vi "WIP_Read_Queue.vi"(8 "error in (no error)":errorcluster, 11 "Queue In":refnum<queue>) -> (0 "error out":errorcluster, 1 "State Out[]":T1[](array[typedef]), 2 "State Out":T1, 3 "Queue out":refnum<queue>)   [LabVIEW 2020]
uses:
  Controls/WIP_State.ctl
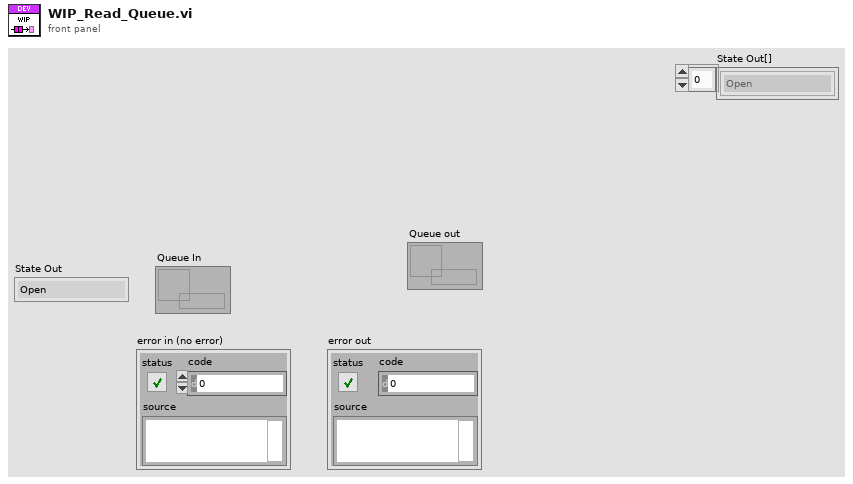
[diagram p1: front panel]
types:
  T1 = typedef "WIP_State.ctl" = enum16{"Open", "Read", "Write", "Read WIP", "Flush", "Close"}
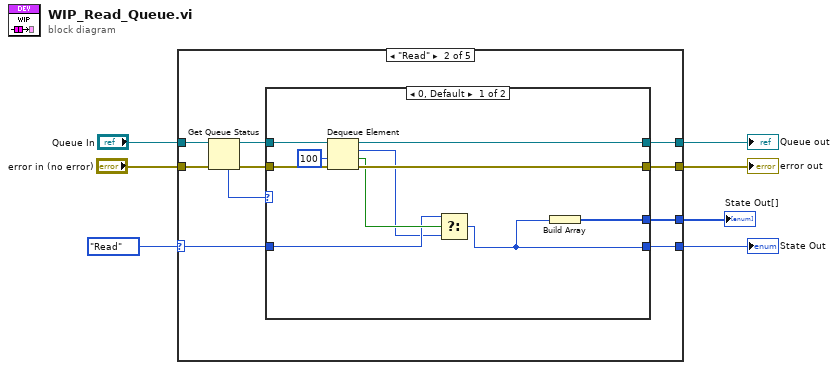
[diagram p0: block diagram]
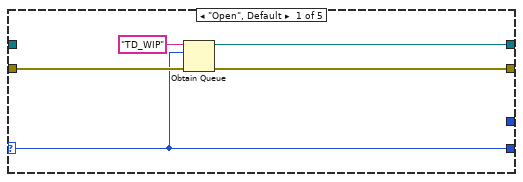
[diagram p2: hidden frame]
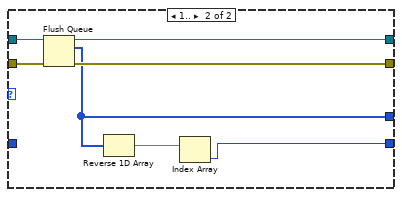
[diagram p3: hidden frame]
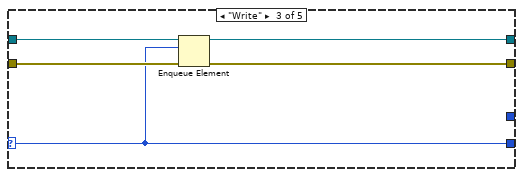
[diagram p4: hidden frame]
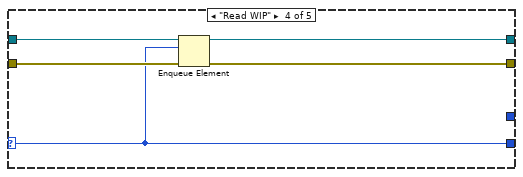
[diagram p5: hidden frame]
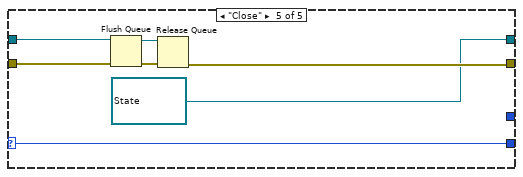
[diagram p6: hidden frame]
diagram:
  n1 = case shown="\"Read\"" WIP_State."Read" ("State In") {
    selector: WIP_State."Read" ("State In") -> [w8 w20 w40 w45 w50]
    tunnel: [w12 w22 w41 w46 w52] -> w7
    tunnel: [w11 w21 w42 w47 w51] -> w6
    tunnel: "error in (no error)" -> [w9 w16 w43 w48 w56]
    tunnel: "Queue In" -> [_ w18 w44 w49 w55]
    tunnel: [w8 w19 w40 w45 w50] -> w2
    tunnel: [_ w13 _ _ _] -> w1
    frame "Open", Default {
      n2 = Obtain Queue(name (unnamed)="TD_WIP", element data type=w8, error in (no error)=w9) -> (queue out=w11:refnum<queue>, error out=w12:errorcluster)  [unwired: 2 in, 1 out]
    }
    frame "Read" {
      n3 = Get Queue Status(queue=w18, error in (no error)=w16) -> (queue out=w17:refnum<queue>, error out=w15:errorcluster, # elements in queue=w14:i32)  [unwired: 1 in, 5 out]
      n4 = case shown="0, Default" w14 {
        tunnel: [w31 w36] -> w22
        tunnel: [w30 w37] -> w21
        tunnel: w20 -> [w28 _]
        tunnel: [w24 w33] -> w19
        tunnel: w17 -> [w26 w39]
        tunnel: w15 -> [w25 w38]
        tunnel: [w23 w35] -> w13
        frame 0, Default {
          n5 = Dequeue Element(queue=w26, timeout in ms (-1)=100, error in (no error)=w25) -> (queue out=w30:refnum<queue>, element=w27:T1, timed out?=w29:bool, error out=w31:errorcluster)
          n6 = Select(t=w28, s=w29, f=w27) -> (s? t:f=w24:T1)
          n7 = Build Array(w24) -> (w23:T1[])
        }
        frame 1.. {
          n8 = Flush Queue(queue=w39, error in (no error)=w38) -> (queue out=w37:refnum<queue>, remaining elements=w35:T1[], error out=w36:errorcluster)
          n9 = Reverse 1D Array(array=w35) -> (reversed array=w34:T1[])
          n10 = Index Array(array=w34) -> (element=w33:T1)  [unwired: 1 in]
        }
      }
    }
    frame "Write" {
      n11 = Enqueue Element(queue=w44, element=w40, error in (no error)=w43) -> (queue out=w42:refnum<queue>, error out=w41:errorcluster)  [unwired: 1 in, 1 out]
    }
    frame "Read WIP" {
      n12 = Enqueue Element(queue=w49, element=w45, error in (no error)=w48) -> (queue out=w47:refnum<queue>, error out=w46:errorcluster)  [unwired: 1 in, 1 out]
    }
    frame "Close" {
      w51 = refnum<queue> refnum items=["Open", "Read", "Write", "Read WIP", "Flush", "Close"] ("Queue In")
      n13 = Flush Queue(queue=w55, error in (no error)=w56) -> (queue out=w53:refnum<queue>, error out=w54:errorcluster)  [unwired: 1 out]
      n14 = Release Queue(queue=w53, error in (no error)=w54) -> (error out=w52:errorcluster)  [unwired: 1 in, 2 out]
    }
  }
  "error out" <- w7
  "Queue out" <- w6
  "State Out" <- w2
  "State Out[]" <- w1
